vi "WriteToStream.vi"(0 "reference in":refnum<class "SuperNS.lvclass">, 2 "LabVIEW Object":T1, 5 "error in":errorcluster, 8 "timeout ms (10000)":i32=10000) -> (14 "reference out":refnum<class "SuperNS.lvclass">, 16 "Write Success":bool, 19 "error out":errorcluster)   [LabVIEW 2020, in "SuperNS.lvclass"]
doc: "Copyright © 2008 - 2024 VI Technologies B.V. \nALL RIGHTS RESERVED\n\nWrite a LabVIEW object to the network stream as a flattened string.\n\nThis will only write if the network stream was successfully created. If an error occurs during write, the <b>Write Success</b> output will be false. The SuperNS object will try and recover the connection internally in the background, but you need to send your data again."
uses:
  SuperNS.lvclass
  StreamDataType.ctl
  SuperNS.lvclass/SuperNS.ctl
panel:
  # "Copyright (c) 2024, VI Technologies B.V.\nAll rights reserved.\n\nRedistribution and use in source and binary forms, with or without modification, are permitted provided that \nthe following conditions are met:\n\n * Redistributions of source code must retain the above copyright notice, this list of conditions and the \nfollowing disclaimer.\n * Redistributions in binary form must reproduce the above copyright notice, this list of conditions and the \nfollowing disclaimer in the documentation and/or other materials provided with the distribution.\n * Neither the name of VI Technologies B.V. nor the names of its contributors may be used to endorse or \npromote products derived from this software without specific prior written permission.\n\nTHIS SOFTWARE IS PROVIDED BY THE COPYRIGHT HOLDERS AND CONTRIBUTORS \"AS IS\" AND ANY EXPRESS OR \nIMPLIED WARRANTIES, INCLUDING, BUT NOT LIMITED TO, THE IMPLIED WARRANTIES OF MERCHANTABILITY \nAND FITNESS FOR A PARTICULAR PURPOSE ARE DISCLAIMED. IN NO EVENT SHALL THE COPYRIGHT OWNER OR \nCONTRIBUTORS BE LIABLE FOR ANY DIRECT, INDIRECT, INCIDENTAL, SPECIAL, EXEMPLARY, OR CONSEQUENTIAL \nDAMAGES (INCLUDING, BUT NOT LIMITED TO, PROCUREMENT OF SUBSTITUTE GOODS OR SERVICES; LOSS OF \nUSE, DATA, OR PROFITS; OR BUSINESS INTERRUPTION) HOWEVER CAUSED AND ON ANY THEORY OF LIABILITY, \nWHETHER IN CONTRACT, STRICT LIABILITY, OR TORT (INCLUDING NEGLIGENCE OR OTHERWISE) ARISING IN ANY \nWAY OUT OF THE USE OF THIS SOFTWARE, EVEN IF ADVISED OF THE POSSIBILITY OF SUCH DAMAGE.\n\nFor more information, please visit https://www.vi-tech.nl or contact us at info@vi-tech.nl"
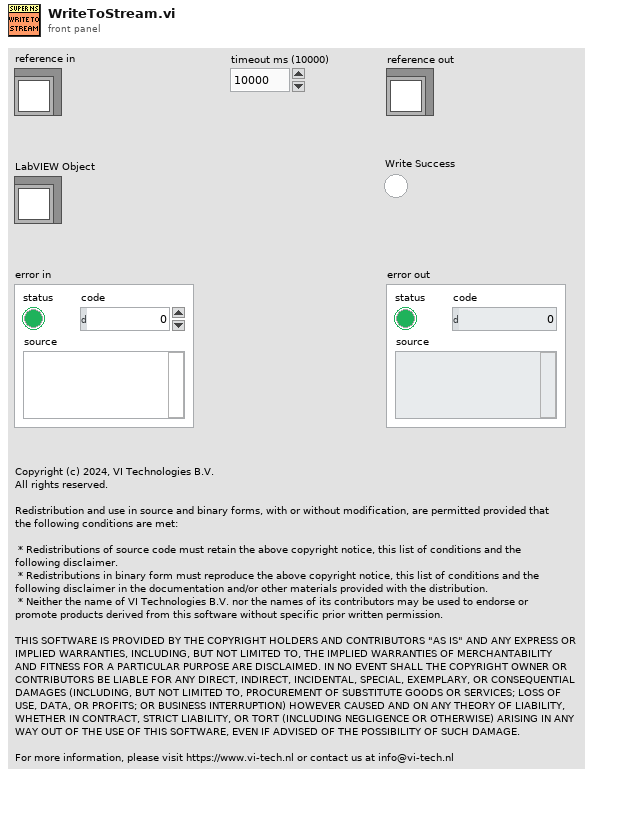
[diagram p1: front panel]
types:
  T1 = typedef "SuperNS.lvclass/StreamDataType.ctl" = refnum<class>
  T2 = typedef "SuperNS.lvclass/ObjectAttributes.ctl" = cluster{"NSName":string, "RemoteEP_URL":string, "BufferSize":i32, "Element Allocation Mode":T3, "ConnLost Timeout":i32, "Writer":bool, "ReadDataEvent":string, "FlushAfterWrite":bool, "Thread":cluster{"VI Refnum":refnum<vi>, "Started Notifier":refnum<notifier>, "Stopped Notifier":refnum<notifier>, "CmdEvent":refnum<user-event>}, "Endpoint":refnum<k21>, "R/W Error":bool, "Flush Wait Condition":T4, "DataReadEvent":refnum<user-event>, "NS Created":bool, "BG ConnCheck/Read period":i32, "ErrorEvent":refnum<user-event>}
  T3 = typedef "Stream Element Allocation Mode.ctl" = u32
  T4 = typedef "Flush And Wait Empty Condition.ctl" = u8
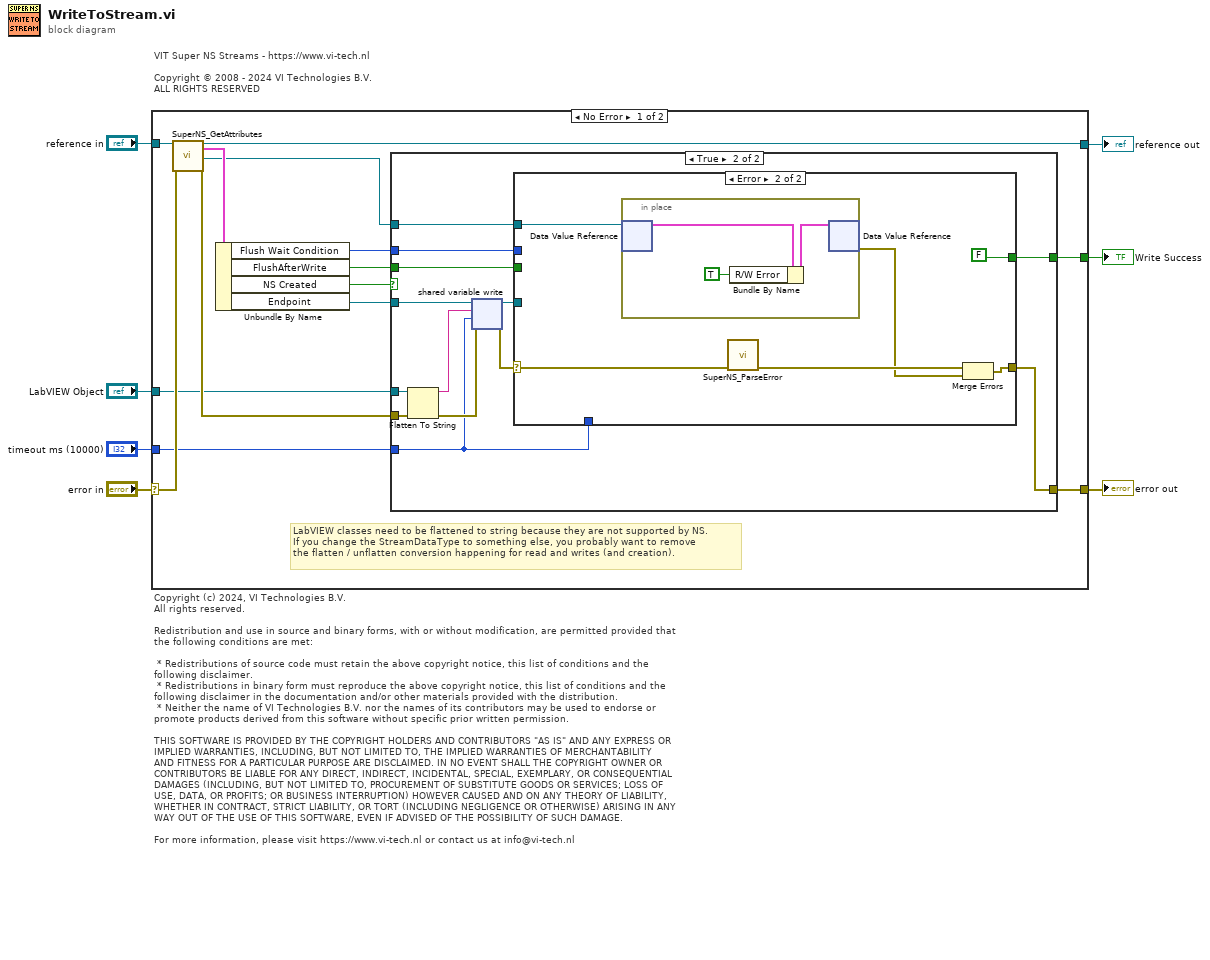
[diagram p0: block diagram]
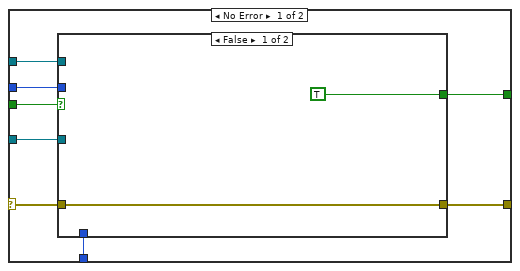
[diagram p3: hidden frame]
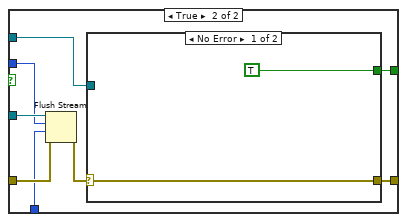
[diagram p4: hidden frame]
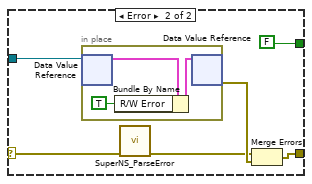
[diagram p5: hidden frame]
diagram:
  # "VIT Super NS Streams - https://www.vi-tech.nl\n\nCopyright © 2008 - 2024 VI Technologies B.V. \nALL RIGHTS RESERVED"
  # "Copyright (c) 2024, VI Technologies B.V.\nAll rights reserved.\n\nRedistribution and use in source and binary forms, with or without modification, are permitted provided that \nthe following conditions are met:\n\n * Redistributions of source code must retain the above copyright notice, this list of conditions and the \nfollowing disclaimer.\n * Redistributions in binary form must reproduce the above copyright notice, this list of conditions and the \nfollowing disclaimer in the documentation and/or other materials provided with the distribution.\n * Neither the name of VI Technologies B.V. nor the names of its contributors may be used to endorse or \npromote products derived from this software without specific prior written permission.\n\nTHIS SOFTWARE IS PROVIDED BY THE COPYRIGHT HOLDERS AND CONTRIBUTORS \"AS IS\" AND ANY EXPRESS OR \nIMPLIED WARRANTIES, INCLUDING, BUT NOT LIMITED TO, THE IMPLIED WARRANTIES OF MERCHANTABILITY \nAND FITNESS FOR A PARTICULAR PURPOSE ARE DISCLAIMED. IN NO EVENT SHALL THE COPYRIGHT OWNER OR \nCONTRIBUTORS BE LIABLE FOR ANY DIRECT, INDIRECT, INCIDENTAL, SPECIAL, EXEMPLARY, OR CONSEQUENTIAL \nDAMAGES (INCLUDING, BUT NOT LIMITED TO, PROCUREMENT OF SUBSTITUTE GOODS OR SERVICES; LOSS OF \nUSE, DATA, OR PROFITS; OR BUSINESS INTERRUPTION) HOWEVER CAUSED AND ON ANY THEORY OF LIABILITY, \nWHETHER IN CONTRACT, STRICT LIABILITY, OR TORT (INCLUDING NEGLIGENCE OR OTHERWISE) ARISING IN ANY \nWAY OUT OF THE USE OF THIS SOFTWARE, EVEN IF ADVISED OF THE POSSIBILITY OF SUCH DAMAGE.\n\nFor more information, please visit https://www.vi-tech.nl or contact us at info@vi-tech.nl"
  n1 = case shown="No Error" "error in" {
    selector: "error in" -> [w21 w75]
    tunnel: [w19 w75] -> w1
    tunnel: [w16 w74] -> w6
    tunnel: "reference in" -> [w18 w74]
    tunnel: "LabVIEW Object" -> [w13 _]
    tunnel: [w11 _] -> w4
    tunnel: "timeout ms (10000)" -> [w8 _]
    frame No Error {
      # "LabVIEW classes need to be flattened to string because they are not supported by NS.\nIf you change the StreamDataType to something else, you probably want to remove\nthe flatten / unflatten conversion happening for read and writes (and creation)."
      n2 = call "SuperNS_GetAttributes.vi"("reference in"=w18, "error in"=w21) -> ("reference out"=w16:refnum<class "SuperNS.lvclass">, "Data"=w17:T2, "DataRef"=w15:refnum<data-value>, "error out"=w20:errorcluster)  [unwired: 14 in]
      n3 = Unbundle By Name(w17) -> ("Flush Wait Condition"=w9:T4, "FlushAfterWrite"=w10:bool, "NS Created"=w12:bool, "Endpoint"=w14:refnum<k21>)
      n4 = case shown="True" w12 {
        tunnel: w15 -> [_ w31]
        tunnel: w14 -> [_ w30]
        tunnel: w13 -> [_ w29]
        tunnel: w20 -> [w22 w35]
        tunnel: [w22 w32] -> w19
        tunnel: [_ w27] -> w11
        tunnel: w10 -> [_ w26]
        tunnel: w9 -> [_ w25]
        tunnel: w8 -> [_ w23]
        frame False {
        }
        frame True {
          n5 = Flatten To String(anything=w29, error in (no error)=w35) -> (data string=w28:string, error out=w34:errorcluster)  [unwired: 2 in, 1 out]
          n6 = shared-variable-write(w30, w34, w28, w23) -> (w24:refnum<k21>, w33:errorcluster)  [unwired: 1 out]
          n7 = case shown="Error" w33 {
            selector: w33 -> [w43 w70]
            tunnel: [w42 w69] -> w32
            tunnel: w31 -> [w36 w66]
            tunnel: [w37 FALSE ("WriteError")] -> w27
            tunnel: w26 -> [w41 _]
            tunnel: w25 -> [w40 _]
            tunnel: w24 -> [w39 _]
            tunnel: w23 -> [w38 _]
            frame No Error {
              n8 = case shown="False" w41 {
                tunnel: w43 -> [w45 w53]
                tunnel: [w45 w51] -> w42
                tunnel: w39 -> [_ w50]
                tunnel: w40 -> [_ w49]
                tunnel: w38 -> [_ w48]
                tunnel: [TRUE ("WriteError") w47] -> w37
                tunnel: w36 -> [_ w46]
                frame False {
                }
                frame True {
                  n9 = Flush Stream(8:w53, 9:w48, 10:w49, 11:w50) -> (0:w52:errorcluster)  [unwired: 2 out]
                  n10 = case shown="No Error" w52 {
                    selector: w52 -> [w55 w61]
                    tunnel: [w55 w59] -> w51
                    tunnel: [TRUE ("WriteError") FALSE ("WriteError")] -> w47
                    tunnel: w46 -> [_ w56]
                    frame No Error {
                    }
                    frame Error {
                      n11 = in-place {
                        n12 = in-place-dvr #1(w56) -> (w63:T2)  [unwired: 1 out]
                        n13 = Bundle By Name(cluster=w63, "R/W Error"=TRUE ("WriteError")) -> (w64:T2)
                        n14 = in-place-dvr #1(w64) -> (w60:errorcluster)  [unwired: 1 out]
                      }
                      n15 = call "SuperNS_ParseError.vi"("error in (no error)"=w61) -> ("error out"=w58:errorcluster)  [unwired: 14 in]
                      n16 = Merge Errors(w58, w60) -> (w59:errorcluster)
                    }
                  }
                }
              }
            }
            frame Error {
              n17 = in-place {
                n18 = in-place-dvr #2(w66) -> (w72:T2)  [unwired: 1 out]
                n19 = Bundle By Name(cluster=w72, "R/W Error"=TRUE ("WriteError")) -> (w71:T2)
                n20 = in-place-dvr #2(w71) -> (w65:errorcluster)  [unwired: 1 out]
              }
              n21 = call "SuperNS_ParseError.vi"("error in (no error)"=w70) -> ("error out"=w68:errorcluster)  [unwired: 14 in]
              n22 = Merge Errors(w68, w65) -> (w69:errorcluster)
            }
          }
        }
      }
    }
    frame Error {
    }
  }
  "reference out" <- w6
  "Write Success" <- w4
  "error out" <- w1
